vi "ConfigInstr.vi"(6 "InstrumentName":string, 7 "VisaRessIn":refnum<visa-resource-name>, 8 "error in (no error)":errorcluster caption="entrée d'erreur (pas d'erreur)", 9 "FirstClassInst":bool, 10 "Function":string, 11 "GenData In":refnum<class "LSCI332.lvclass"> caption="DNL_LabVIEW Object in") -> (0 "error out":errorcluster caption="sortie d'erreur", 3 "GenData Out":refnum<class "LSCI332.lvclass"> caption="DNL_LabVIEW Object out")   [LabVIEW 2019, in "LSCI332.lvclass"]
uses:
  LSCI332.lvclass
  C:/Programmes Labview/LabScanV1A/DevicesClass/BaseDevice/BaseDevice.lvclass
  LSCI332_Func.ctl
  LSCI332.lvclass/LSCI332.ctl
  BaseDevice/BaseDevice.lvclass/BaseDevice.ctl
  BaseDevice/Accessor/SetShowInstrNm.vi
  BaseDevice/Accessor/SetInstrParam.vi
panel:
  in  "Class_Func":T1
  out "VisaRessOut":refnum<visa-resource-name>
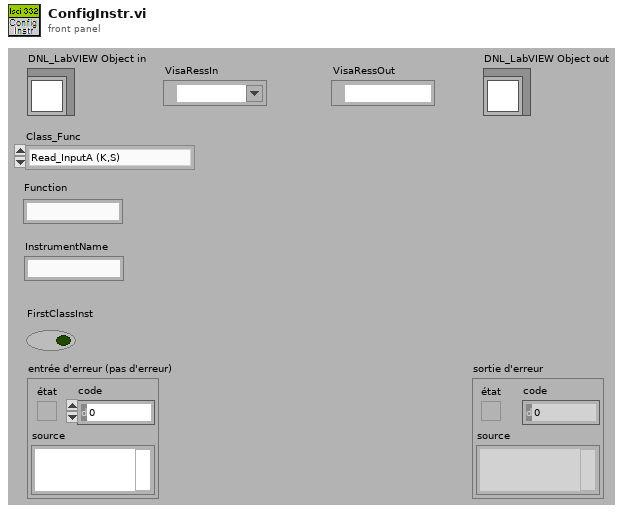
[diagram p1: front panel]
types:
  T1 = typedef "LSCI332.lvclass/LSCI332_Func.ctl" = enum16{"Read_InputA (K,S)", "Read_InputA&Heater (K,S,%,W)", "Read_InputB (K,S)", "Read_InputB&Heater (K,S,%,W)", "Read_Heater (%,W)", "Read_InputA&B(K,S,K,S)", "Read_InputA&B&Heater (K,S,K,S,%,W)", "Scan_Loop1 (K,S)", "Scan_Loop2(K,S)", "Util (na)"}
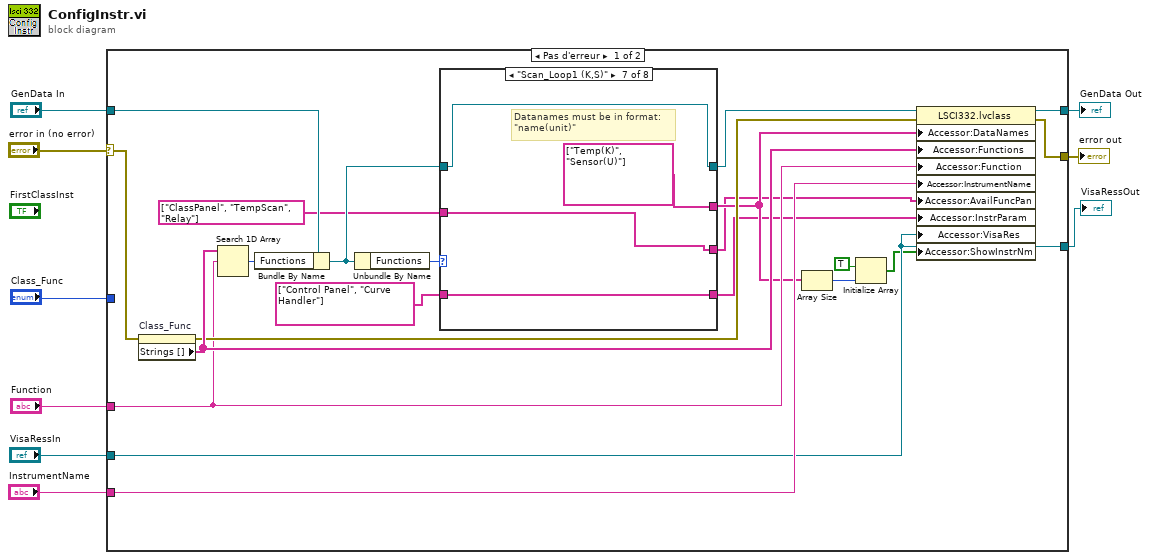
[diagram p0: block diagram]
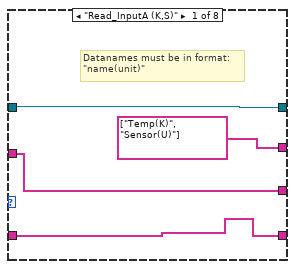
[diagram p2: hidden frame]
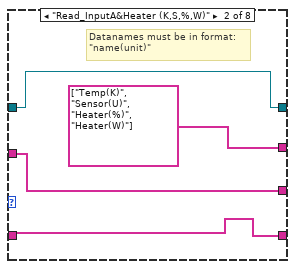
[diagram p3: hidden frame]
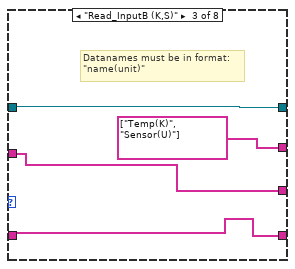
[diagram p4: hidden frame]
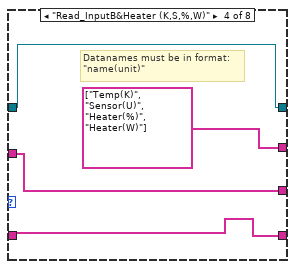
[diagram p5: hidden frame]
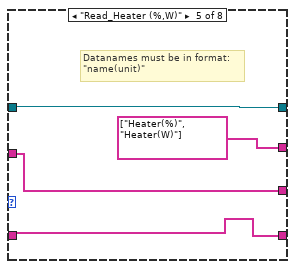
[diagram p6: hidden frame]
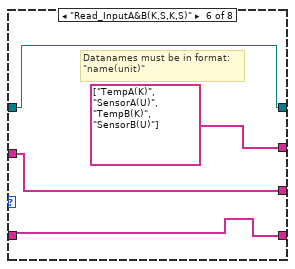
[diagram p7: hidden frame]
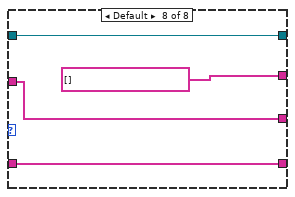
[diagram p8: hidden frame]
diagram:
  n1 = case shown="Pas d'erreur" "error in (no error)" {
    selector: "error in (no error)" -> [w24 w64]
    tunnel: [w30 w64] -> w8
    tunnel: "GenData In" -> [w25 w63]
    tunnel: [w29 w63] -> w6
    tunnel: "Class_Func" -> [_ _]
    tunnel: "Function" -> [w20 _]
    tunnel: "InstrumentName" -> [w19 _]
    tunnel: "VisaRessIn" -> [w18 _]
    tunnel: [w18 _] -> w1
    frame No Error {
      n2 = property on="Class_Func" class="Énum (strict)"(error in=w24) -> (error out=w23:errorcluster, "Strings []"=w27:string[])  [unwired: 1 in, 1 out]
      n3 = Search 1D Array(1D array=w27, element=w20) -> (index of element=w26:i32)  [unwired: 1 in]
      n4 = Bundle By Name(cluster=w25, "Functions"=w26) -> (w22:refnum<class "LSCI332.lvclass">)
      n5 = Unbundle By Name(w22) -> ("Functions"=w28:T1)
      n6 = case shown="\"Scan_Loop1 (K,S)\"" w28 {
        tunnel: [string[] ["Temp(K)", "Sensor(U)"] string[] ["Temp(K)", "Sensor(U)", "Heater(%)", "Heater(W)"] string[] ["Temp(K)", "Sensor(U)"] string[] ["Temp(K)", "Sensor(U)", "Heater(%)", "Heater(W)"] string[] ["Heater(%)", "Heater(W)"] string[] ["TempA(K)", "SensorA(U)", "TempB(K)", "SensorB(U)"] string[] ["Temp(K)", "Sensor(U)"] string[] []] -> w15
        tunnel: w22 -> [w34 w37 w42 w46 w50 w54 w58 w62]
        tunnel: [w34 w37 w42 w46 w50 w54 w58 w62] -> w21
        tunnel: [w32 w36 w40 w44 w48 w52 w56 w61] -> w12
        tunnel: [w31 w35 w39 w43 w47 w51 w55 w59] -> w10
        tunnel: string[] ["ClassPanel", "TempScan", "Relay"] -> [w32 w36 w40 w44 w48 w52 w56 w61]
        tunnel: string[] ["Control Panel", "Curve Handler"] -> [w31 w35 w39 w43 w47 w51 w55 w59]
        frame "Read_InputA (K,S)" {
          # "Datanames must be in format:\n\"name(unit)\""
        }
        frame "Read_InputA&Heater (K,S,%,W)" {
          # "Datanames must be in format:\n\"name(unit)\""
        }
        frame "Read_InputB (K,S)" {
          # "Datanames must be in format:\n\"name(unit)\""
        }
        frame "Read_InputB&Heater (K,S,%,W)" {
          # "Datanames must be in format:\n\"name(unit)\""
        }
        frame "Read_Heater (%,W)" {
          # "Datanames must be in format:\n\"name(unit)\""
        }
        frame "Read_InputA&B(K,S,K,S)" {
          # "Datanames must be in format:\n\"name(unit)\""
        }
        frame "Scan_Loop1 (K,S)" {
          # "Datanames must be in format:\n\"name(unit)\""
        }
        frame Default {
        }
      }
      n7 = Array Size(array=w15) -> (size(s)=w17:i32)
      n8 = Initialize Array(TRUE, w17) -> (w14:bool[])
      n9 = property class="LSCI332.lvclass"(reference=w21, error in=w23, "Accessor:DataNames"=w15, "Accessor:Functions"=w27, "Accessor:Function"=w20, "Accessor:InstrumentName"=w19, "Accessor:AvailFuncPan"=w12, "Accessor:InstrParam"=w10, "Accessor:VisaRes"=w18, "Accessor:ShowInstrNm"=w14) -> (reference out=w29:refnum<class "LSCI332.lvclass">, error out=w30:errorcluster)
    }
    frame Error {
    }
  }
  "error out" <- w8
  "GenData Out" <- w6
  "VisaRessOut" <- w1
